vi "Write User File (SubVI).vi"(0 "configuration file path":path=path "C:/Projet_CETAL_DESY_CSCI/POSTES LOCAUX/PROJECT_GAIA_HP/Development/Config/User.ini" caption="chemin du fichier de configuration", 1 "User file contents Energie UV":dbl[](array[numeric]) format="%#.3g", 2 "User file contents Puissance depolar":dbl[](array[numeric]) format="%#.3g", 3 "User file contents Energie IR":dbl[](array[numeric]) format="%#.3g", 7 "error in (no error)":errorcluster caption="entrée d'erreur (pas d'erreur)") -> (24 "error?":bool caption="erreur ?", 27 "error out":errorcluster caption="sortie d'erreur")   [LabVIEW 2017]
doc: "by Tanguy BOULARD"
uses:
  <vilib>/Utility/config.llb/Write Key (String).vi
  <vilib>/Utility/config.llb/NI_LVConfig.lvlib
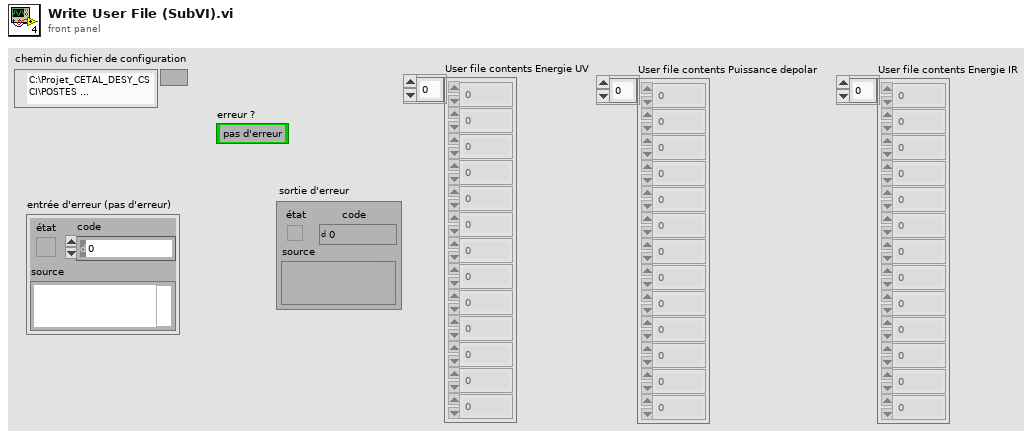
[diagram p1: front panel]
types:
  T1 = typedef "NI_LVConfig.lvlib/Config Data RefNum.ctl" = refnum<k1>
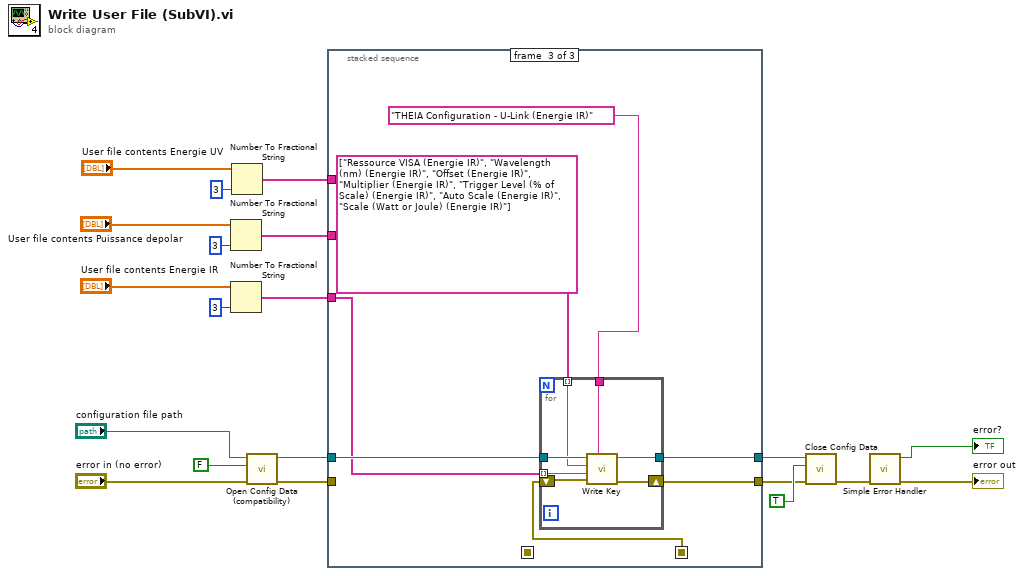
[diagram p0: block diagram]
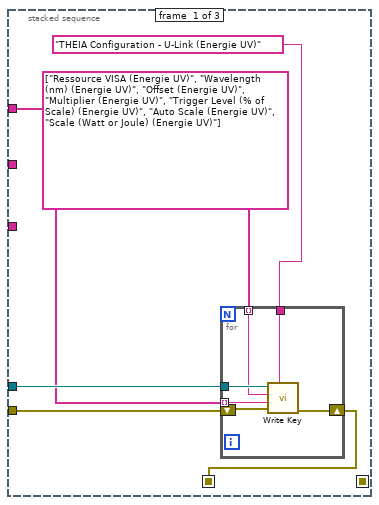
[diagram p2: hidden frame]
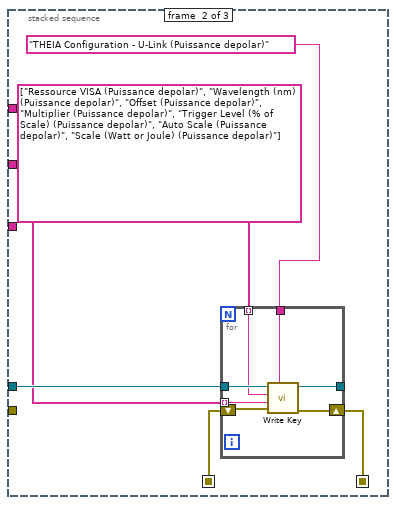
[diagram p3: hidden frame]
diagram:
  n1 = Number To Fractional String(number="User file contents Puissance depolar", precision (6)=i16 3) -> (F-format string=w2:string[])  [unwired: 2 in]
  n2 = Number To Fractional String(number="User file contents Energie IR", precision (6)=i16 3) -> (F-format string=w1:string[])  [unwired: 2 in]
  n3 = Number To Fractional String(number="User file contents Energie UV", precision (6)=i16 3) -> (F-format string=w8:string[])  [unwired: 2 in]
  n4 = call <vilib>:"Open Config Data (compatibility).vi"("error in (no error)"="error in (no error)", "create file if necessary (T)"=FALSE ("create file if necessary? (T)"), "configuration file path"="configuration file path") -> ("error out"=w19:errorcluster, "refnum"=w14:T1)  [unwired: 6 in, 1 out]
  n5 = stacked-sequence {
    seq-local: [w21 _ _] -> [_ w34 _]
    seq-local: [_ w33 _] -> [_ _ w46]
    tunnel: w19 -> [w26 _ _]
    tunnel: w14 -> [w25 w38 w52]
    tunnel: [_ _ w51] -> w11
    tunnel: [_ _ w50] -> w10
    tunnel: w8 -> [w24 _ _]
    tunnel: w2 -> [_ w35 _]
    tunnel: w1 -> [_ _ w47]
    frame #0 {
      n6 = for {
        shift-right: [w31] -> w21
        shift-left: w26 -> [w32]
        tunnel: w25 -> [w30]
        tunnel: w24 -> [w29] mode=indexing
        tunnel: string[] ["Ressource VISA (Energie UV)", "Wavelength (nm) (Energie UV)", "Offset (Energie UV)", "Multiplier (Energie UV)", "Trigger Level (% of Scale) (Energie UV)", "Auto Scale (Energie UV)", "Scale (Watt or Joule) (Energie UV)"] -> [w28] mode=indexing
        tunnel: "THEIA Configuration - U-Link (Energie UV)" ("section") -> [w27]
        n7 = call-poly <vilib>:"Write Key.vi"("section"=w27, "error in (no error)"=w32, "value"=w29, "key"=w28, "refnum"=w30) -> ("error out"=w31:errorcluster)  [unwired: 4 in, 2 out]
      }
    }
    frame #1 {
      n8 = for {
        shift-right: [w44] -> w33
        shift-left: w34 -> [w45]
        tunnel: w38 -> [w43]
        tunnel: w35 -> [w42] mode=indexing
        tunnel: [w41] -> _
        tunnel: string[] ["Ressource VISA (Puissance depolar)", "Wavelength (nm) (Puissance depolar)", "Offset (Puissance depolar)", "Multiplier (Puissance depolar)", "Trigger Level (% of Scale) (Puissance depolar)", "Auto Scale (Puissance depolar)", "Scale (Watt or Joule) (Puissance depolar)"] -> [w40] mode=indexing
        tunnel: "THEIA Configuration - U-Link (Puissance depolar)" ("section") -> [w39]
        n9 = call-poly <vilib>:"Write Key.vi"("section"=w39, "error in (no error)"=w45, "value"=w42, "key"=w40, "refnum"=w43) -> ("error out"=w44:errorcluster, "refnum out"=w41:T1)  [unwired: 4 in, 1 out]
      }
    }
    frame #2 {
      n10 = for {
        shift-right: [w58] -> w51
        shift-left: w46 -> [w59]
        tunnel: w52 -> [w57]
        tunnel: w47 -> [w56] mode=indexing
        tunnel: [w55] -> w50
        tunnel: string[] ["Ressource VISA (Energie IR)", "Wavelength (nm) (Energie IR)", "Offset (Energie IR)", "Multiplier (Energie IR)", "Trigger Level (% of Scale) (Energie IR)", "Auto Scale (Energie IR)", "Scale (Watt or Joule) (Energie IR)"] -> [w54] mode=indexing
        tunnel: "THEIA Configuration - U-Link (Energie IR)" ("section") -> [w53]
        n11 = call-poly <vilib>:"Write Key.vi"("section"=w53, "error in (no error)"=w59, "value"=w56, "key"=w54, "refnum"=w57) -> ("error out"=w58:errorcluster, "refnum out"=w55:T1)  [unwired: 4 in, 1 out]
      }
    }
  }
  n12 = call <vilib>:"Close Config Data.vi"("error in (no error)"=w11, "write file if changed (T)"=TRUE ("write configuration file? (T)"), "refnum"=w10) -> ("error out"=w18:errorcluster)  [unwired: 8 out]
  n13 = call <vilib>:"Simple Error Handler.vi"("error in (no error)"=w18) -> ("error?"=→"error?":bool, "error out"=→"error out":errorcluster)  [unwired: 1 in, 6 out]
